vi "Datatype Comparision.vi"(2 "Required Datatype":T1, 3 "Data":variant) -> (0 "Null?":bool, 1 "Equal?":bool)   [LabVIEW 2016]
uses:
  Datatype.ctl
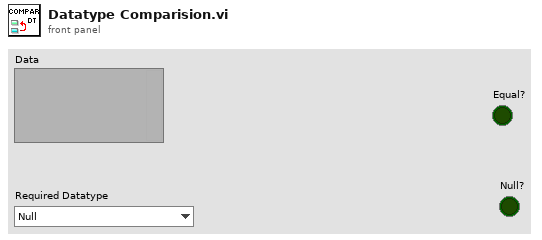
[diagram p1: front panel]
types:
  T1 = typedef "Datatype.ctl" = enum16{"Null", "Numeric", "String", "Bool", "Numeric 1D", "String 1D", "Bool 1D", "Numeric 2D", "String 2D", "Bool 2D", "Variant"}
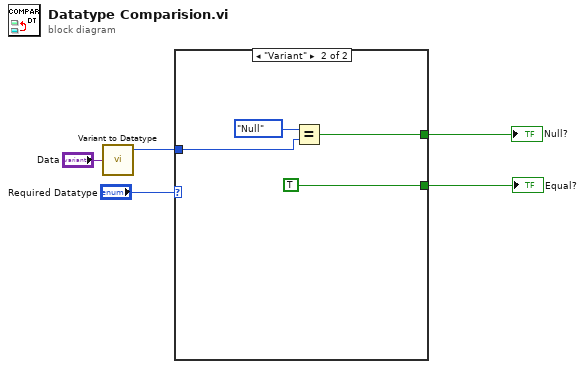
[diagram p0: block diagram]
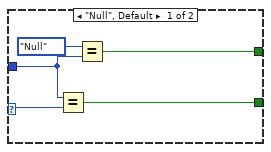
[diagram p2: hidden frame]
diagram:
  n1 = call "Variant to Datatype.vi"("Variant"="Data") -> ("Datatype"=w3:T1)  [unwired: 2 in, 2 out]
  n2 = case shown="\"Variant\"" "Required Datatype" {
    selector: "Required Datatype" -> [w10 _]
    tunnel: w3 -> [w8 w12]
    tunnel: [w9 TRUE] -> w4
    tunnel: [w6 w11] -> w1
    frame "Null", Default {
      n3 = Equal?(x=w8, y=w10) -> (x = y?=w9:bool)
      n4 = Equal?(x=Datatype."Null", y=w8) -> (x = y?=w6:bool)
    }
    frame "Variant" {
      n5 = Equal?(x=Datatype."Null", y=w12) -> (x = y?=w11:bool)
    }
  }
  "Equal?" <- w4
  "Null?" <- w1
